vi "Read Holding Regs.vi"(0 "reference in":refnum<class "MB_MODULE.lvclass">, 5 "starting address":u16, 7 "number of inputs":u16, 11 "error in (no error)":errorcluster) -> (4 "register values":u16[](array[numeric]), 15 "error out":errorcluster)   [LabVIEW 2019, in "MB_MODULE.lvclass"]
uses:
  MB_MODULE.lvclass
  MB_MODULE.lvclass/MB_MODULE.ctl
  <vilib>/NI/Modbus Library/API/Master/Modbus Master.lvclass
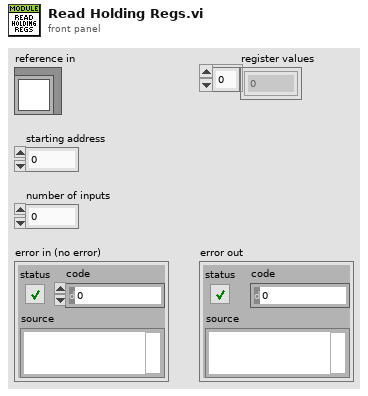
[diagram p1: front panel]
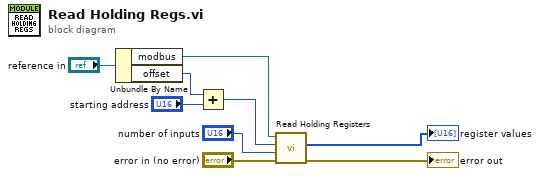
[diagram p0: block diagram]
diagram:
  n1 = Unbundle By Name("reference in") -> ("modbus"=w2:refnum<class "Modbus Master.lvclass">, "offset"=w6:u16)
  n2 = Add(x=w6, y="starting address") -> (x+y=w5:u16)
  n3 = call-dynamic "Read Holding Registers.vi"("error in"="error in (no error)", "number of inputs"="number of inputs", "starting address"=w5, "Modbus master in"=w2) -> ("error out"=→"error out":errorcluster, "register values"=→"register values":u16[])  [unwired: 5 in, 1 out]
